vi "Model - Get Stop.vi"(8 "error in (no error)":errorcluster, 11 "View Model":T1) -> (0 "error out":errorcluster, 2 "Stop?":bool, 3 "View Model":T1)   [LabVIEW 2017]
doc: "Get actual Stop value from DVR"
uses:
  Controls/View Model.ctl
  Controls/Shared Model.ctl
  Error Handler/Controls/Error Model.ctl
  Error Handler/Controls/Error Event.ctl
  Error Handler/Controls/Error Type.ctl
  Controller/Controls/Controller Model.ctl
  Controller/Controls/Controller Event.ctl
  Controller/Controls/Controller Command.ctl
  Controller/Controls/Controller Overhead.ctl
  Real-Time/RT Status.ctl
  Real-Time/RT Loop Status.ctl
  Controller/Controls/Controller NStream.ctl
  Controller/Controls/Controller DAQ Data.ctl
  TDMS Logger/Controls/TDMS Model.ctl
  TDMS Logger/Controls/TDMS Event.ctl
  TDMS Logger/Controls/TDMS Command.ctl
  TDMS Logger/Controls/TDMS Overhead.ctl
  TDMS Logger/Controls/TDMS ChanProperties.ctl
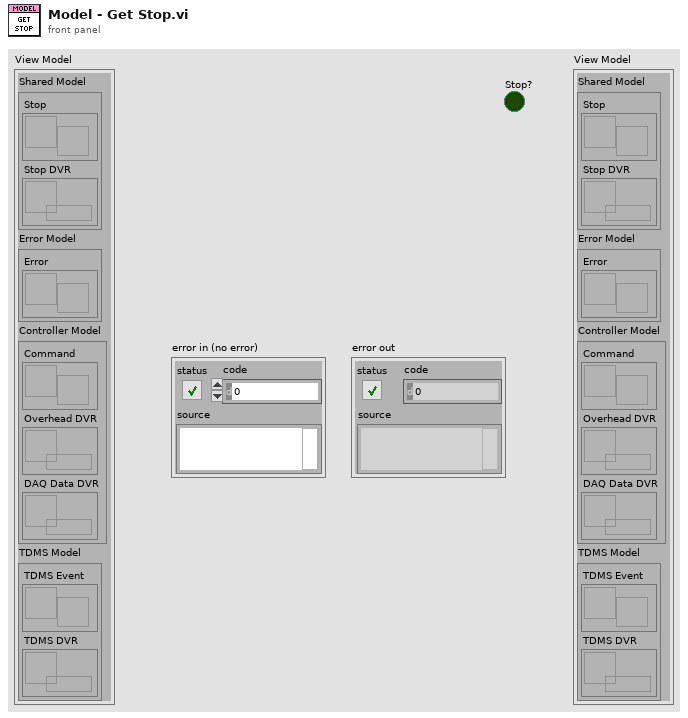
[diagram p1: front panel]
types:
  T1 = typedef "View Model.ctl" = cluster{"Shared Model":T2, "Error Model":T3, "Controller Model":T4, "TDMS Model":T5}
  T2 = typedef "Shared Model.ctl" = cluster{"Stop":refnum<user-event>, "Stop DVR":refnum<data-value>}
  T3 = typedef "Error Model.ctl" = cluster{"Error":refnum<user-event>}
  T4 = typedef "Controller Model.ctl" = cluster{"Command":refnum<user-event>, "Overhead DVR":refnum<data-value>, "DAQ Data DVR":refnum<data-value>}
  T5 = typedef "TDMS Model.ctl" = cluster{"TDMS Event":refnum<user-event>, "TDMS DVR":refnum<data-value>}
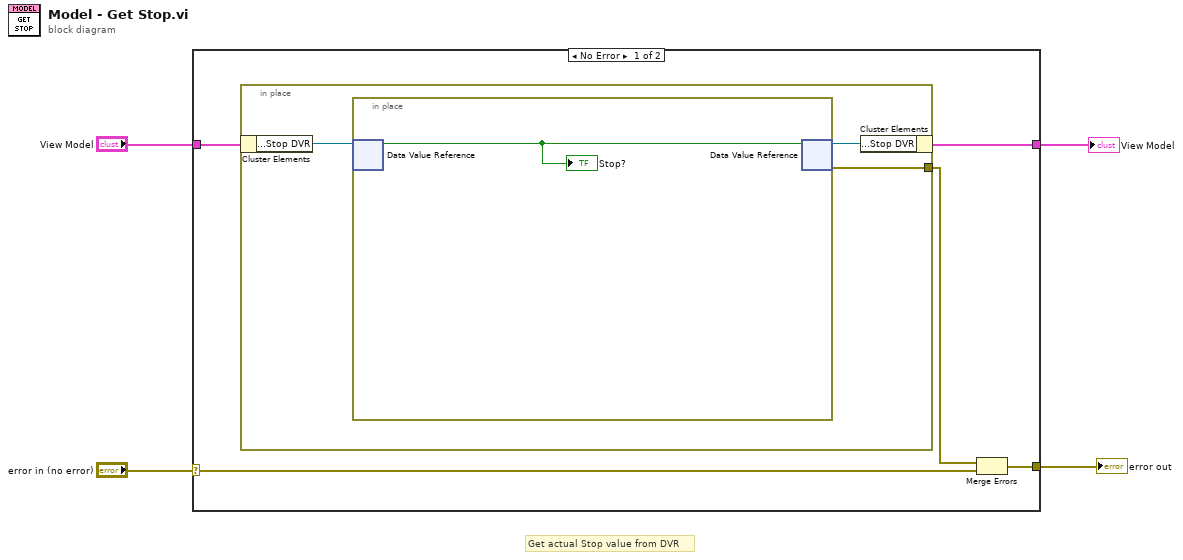
[diagram p0: block diagram]
diagram:
  # "Get actual Stop value from DVR"
  n1 = case shown="No Error" "error in (no error)" {
    selector: "error in (no error)" -> [w6 w14]
    tunnel: "View Model" -> [w9 w15]
    tunnel: [w8 w15] -> w2
    tunnel: [w5 w14] -> w1
    frame No Error {
      n2 = in-place {
        in-place-border: [w10] -> w7
        n3 = in-place-cluster #1(w9) -> ("Shared Model.Stop DVR"=w12:refnum<data-value>)
        n4 = in-place {
          n5 = in-place-dvr #2(w12) -> (w13:bool)  [unwired: 1 out]
          "Stop?" <- w13
          n6 = in-place-dvr #2(w13) -> (w11:refnum<data-value>, w10:errorcluster)
        }
        n7 = in-place-cluster #1("Shared Model.Stop DVR"=w11) -> (w8:T1)
      }
      n8 = Merge Errors(w7, w6) -> (w5:errorcluster)
    }
    frame Error {
    }
  }
  "View Model" <- w2
  "error out" <- w1
